vi "Get Grid Position.vi"(2 "Position In":refnum<class "Vector2.lvclass">, 3 "Collision Grid in":refnum<class "CollisionGrid.lvclass">) -> (0 "grid y out":i16, 1 "grid x out":i16)   [LabVIEW 2022 SP3, in "CollisionGrid.lvclass"]
uses:
  CollisionGrid.lvclass
  Math/Vector2/Vector2.lvclass
  CollisionGrid.lvclass/CollisionGrid.ctl
  Math/Vector2/Vector2.lvclass/Vector2.ctl
  Math/Vector2/Read x.vi
  Math/Vector2/Read y.vi
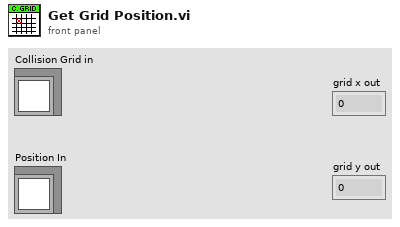
[diagram p1: front panel]
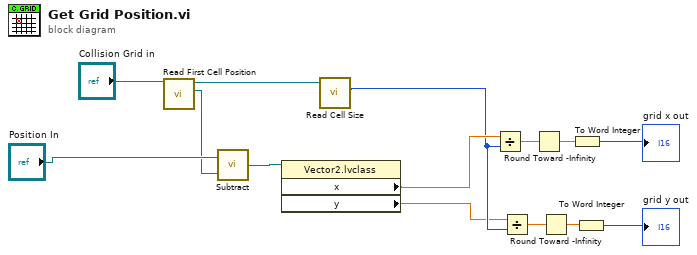
[diagram p0: block diagram]
diagram:
  n1 = call "Read First Cell Position.vi"("CollisionGrid in"="Collision Grid in") -> ("First Cell Position out"=w2:refnum<class "Vector2.lvclass">, "CollisionGrid out"=w5:refnum<class "CollisionGrid.lvclass">)  [unwired: 8 in, 1 out]
  n2 = call "Subtract.vi"("Vec2 b in"=w2, "Vec2 a in"="Position In") -> ("Vec2 out"=w4:refnum<class "Vector2.lvclass">)
  n3 = property class="Vector2.lvclass"(reference=w4) -> ("x"=w8:sgl, "y"=w1:sgl)  [unwired: 1 in, 2 out]
  n4 = call "Read Cell Size.vi"("CollisionGrid in"=w5) -> ("Cell Size"=w7:i16)  [unwired: 8 in, 2 out]
  n5 = Divide(x=w8, y=w7) -> (x/y=w14:sgl)
  n6 = Divide(x=w1, y=w7) -> (x/y=w13:sgl)
  n7 = Round Toward -Infinity(1:w14) -> (0:w11:sgl)
  n8 = Round Toward -Infinity(1:w13) -> (0:w12:sgl)
  n9 = To Word Integer(number=w11) -> (16bit integer=→"grid x out":i16)
  n10 = To Word Integer(number=w12) -> (16bit integer=→"grid y out":i16)
